vi "GPS Example.vi"() -> ()   [LabVIEW 2012, in "Phidget GPS.lvlib"]
uses:
  <instrlib>/Phidgets/Phidget GPS/Phidget GPS.lvlib
  <instrlib>/Phidgets/Phidget GPS/Public/GPSStart.vi
  <instrlib>/Phidgets/Phidget GPS/Public/GPSClose.vi
  <instrlib>/Phidgets/Phidget Common/Phidget Common.lvlib
panel:
  out "Latitude":dbl
  out "Heading":dbl
  out "Date":T1
  out "Altitude":dbl
  out "Velocity":dbl
  out "Time":T2
  out "PositionFixState":bool
  out "Longitude":dbl
  out "error out":errorcluster
  in  "error in (no error)":errorcluster
  in  "Device Info":T3={"Serial Number"=-1, "Channel"=0, "Port"=0}
  out "Attached?":bool
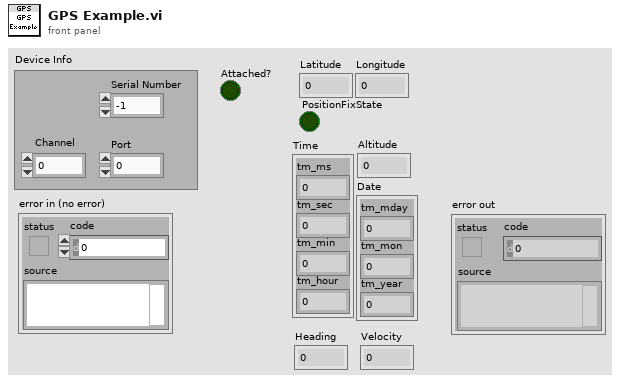
[diagram p1: front panel]
types:
  T1 = cluster{"tm_mday":i16, "tm_mon":i16, "tm_year":i16}
  T2 = cluster{"tm_ms":i16, "tm_sec":i16, "tm_min":i16, "tm_hour":i16}
  T3 = cluster{"Serial Number":i32, "Channel":i32, "Port":i32}
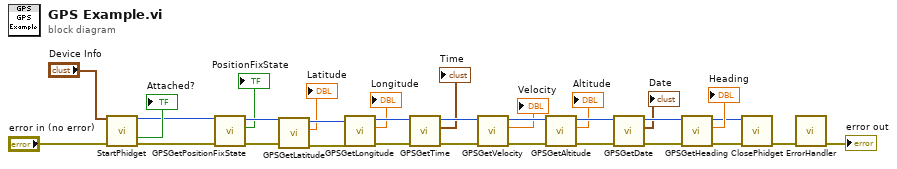
[diagram p0: block diagram]
diagram:
  n1 = call-poly <instrlib>:"StartPhidget.vi"("Device Info"="Device Info", "error in (no error)"="error in (no error)") -> ("Phidget ID"=w2:u64, "Attached?"=→"Attached?":bool, "error out"=w3:errorcluster)  [unwired: 10 in, 1 out]
  n2 = call <instrlib>:"GPSGetPositionFixState.vi"("error in (no error)"=w3, "Device In"=w2) -> ("error out"=w20:errorcluster, "PositionFixState"=→"PositionFixState":bool, "Device Out"=w13:u64)  [unwired: 6 in]
  n3 = call <instrlib>:"GPSGetLatitude.vi"("error in (no error)"=w20, "Device In"=w13) -> ("error out"=w21:errorcluster, "Latitude"=→"Latitude":dbl, "Device Out"=w14:u64)  [unwired: 6 in]
  n4 = call <instrlib>:"GPSGetLongitude.vi"("error in (no error)"=w21, "Device In"=w14) -> ("error out"=w22:errorcluster, "Longitude"=→"Longitude":dbl, "Device Out"=w15:u64)  [unwired: 6 in]
  n5 = call <instrlib>:"GPSGetTime.vi"("error in (no error)"=w22, "Device In"=w15) -> ("error out"=w23:errorcluster, "Time"=→"Time":T2, "Device Out"=w16:u64)  [unwired: 6 in]
  n6 = call <instrlib>:"GPSGetVelocity.vi"("error in (no error)"=w23, "Device In"=w16) -> ("error out"=w24:errorcluster, "Velocity"=→"Velocity":dbl, "Device Out"=w17:u64)  [unwired: 6 in]
  n7 = call <instrlib>:"GPSGetAltitude.vi"("error in (no error)"=w24, "Device In"=w17) -> ("error out"=w25:errorcluster, "Altitude"=→"Altitude":dbl, "Device Out"=w18:u64)  [unwired: 6 in]
  n8 = call <instrlib>:"GPSGetDate.vi"("error in (no error)"=w25, "Device In"=w18) -> ("error out"=w26:errorcluster, "Date"=→"Date":T1, "Device Out"=w19:u64)  [unwired: 6 in]
  n9 = call <instrlib>:"GPSGetHeading.vi"("error in (no error)"=w26, "Device In"=w19) -> ("error out"=w1:errorcluster, "Heading"=→"Heading":dbl, "Device Out"=w4:u64)  [unwired: 6 in]
  n10 = call-poly <instrlib>:"ClosePhidget.vi"("error in"=w1, "Device In"=w4) -> ("error out"=w28:errorcluster)  [unwired: 9 in]
  n11 = call <instrlib>:"ErrorHandler.vi"("error in"=w28) -> ("error out"=→"error out":errorcluster)  [unwired: 9 in, 1 out]
